vi "createActuator.vi"(8 "error in (no error)":errorcluster, 10 "Actuator Types":T1, 11 "IActuatorFactory in":refnum<class "ActuatorFactory.lvclass">) -> (0 "error out":errorcluster, 2 "Actuator":refnum<class "IActuator.lvclass">, 3 "IActuatorFactory out":refnum<class "ActuatorFactory.lvclass">)   [LabVIEW 2015, in "ActuatorFactory.lvclass"]
uses:
  ActuatorFactory.lvclass
  IActuator/IActuator.lvclass
  Typedefs/Actuator Types.ctl
  Typedefs/Pressure Servo Settings.ctl
  Typedefs/ClosedLoopSettings.ctl
  Typedefs/Flow Control Settings.ctl
  Typedefs/DAC Settings.ctl
  Calculators/VoltageToILCDACRaw/VoltageToILCDACRaw.lvclass
  ActuatorCylinder/ILCControlledActuatorCylinder/ILCControlledActuatorCylinder.lvclass
  ILCDACFactory/ILCDACFactory/ILCDACFactory.lvclass
  Calculators/VoltageToILCDACRaw/VoltageToILCDACRaw.lvclass/VoltageToILCDACRaw.ctl
  ActuatorCylinder/ILCControlledActuatorCylinder/ILCControlledActuatorCylinder.lvclass/ILCControlledActuatorCylinder.ctl
  SingleCylinderActuator/SingleCylinderActuator.lvclass
  SingleCylinderActuator/SingleCylinderActuator.lvclass/SingleCylinderActuator.ctl
  ConfigurationTestParameters/ConfigurationTestParameters.lvclass
  Typedefs/FAMTTypedefs.lvlib
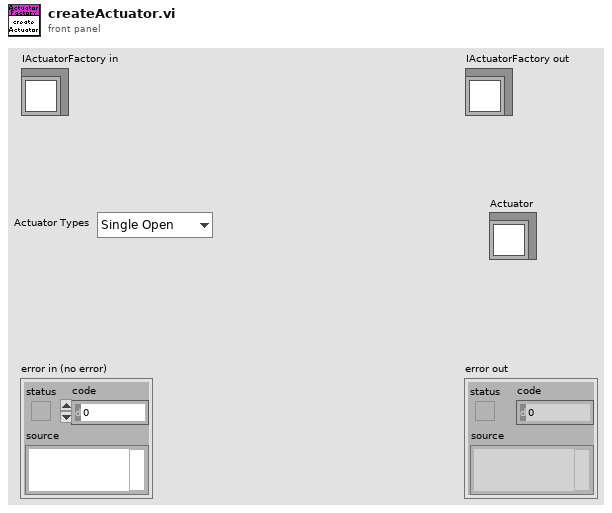
[diagram p1: front panel]
types:
  T1 = typedef "FAMTTypedefs.lvlib/Actuator Types.ctl" = enum16{"Single Open"}
  T2 = typedef "FAMTTypedefs.lvlib/DAC Settings.ctl" = cluster{"Voltage Reference":dbl[unit], "Min Counts":i32, "Max Counts":i32}
  T3 = typedef "FAMTTypedefs.lvlib/Flow Control Settings.ctl" = cluster{"DAC Channel":u8, "ROT Bias":u8, "Minimum Voltage":dbl, "Maximum Voltage":dbl, "Off Value":dbl}
  T4 = typedef "FAMTTypedefs.lvlib/Pressure Servo Settings.ctl" = cluster{"Center Point":dbl[unit], "Area":dbl, "PA to PSI":dbl, "Servo 1 DAC Channel":u8, "Servo 2 DAC Channel":u8, "Closed Loop Settings":T5, "Off Value":dbl}
  T5 = typedef "FAMTTypedefs.lvlib/ClosedLoopSettings.ctl" = cluster{"P":dbl, "I":dbl, "D":dbl, "Minimum":dbl, "Maximum":dbl}
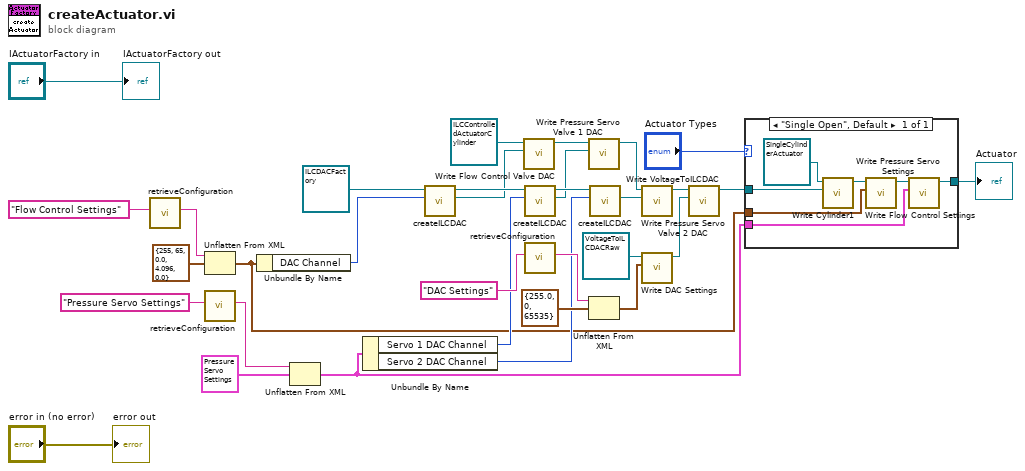
[diagram p0: block diagram]
diagram:
  n1 = call "retrieveConfiguration.vi"("configName"="Flow Control Settings") -> ("xmlConfig"=w25:string)  [unwired: 8 in, 2 out]
  n2 = Unflatten From XML(xml string=w25, type=T3 {"DAC Channel"=255, "ROT Bias"=65, "Minimum Voltage"=0.0, "Maximum Voltage"=4.096, "Off Value"=0.0} ("Flow Control Settings")) -> (value=w1:T3)  [unwired: 1 in, 1 out]
  n3 = call "retrieveConfiguration.vi"("configName"="Pressure Servo Settings") -> ("xmlConfig"=w28:string)  [unwired: 8 in, 2 out]
  n4 = Unbundle By Name(w1) -> ("DAC Channel"=w6:u8)
  n5 = Unflatten From XML(xml string=w28, type=T4 {"Center Point"=413685.4733709468, "Area"=0.004536, "PA to PSI"=0.000145038, "Servo 1 DAC Channel"=1, "Servo 2 DAC Channel"=2, "Closed Loop Settings"={"P"=1.0, "I"=0.1, "D"=0.0, "Minimum"=0.0, "Maximum"=10.0}, "Off Value"=0.004536} ("Pressure Servo Settings")) -> (value=w4:T4)  [unwired: 1 in, 1 out]
  n6 = Unbundle By Name(w4) -> ("Servo 1 DAC Channel"=w15:u8, "Servo 2 DAC Channel"=w14:u8)
  n7 = call-dynamic "createILCDAC.vi"("Channel"=w6, "ILCDACFactory in"=refnum<class "ILCDACFactory.lvclass"> refnum ("ILCDACFactory.lvclass")) -> ("ILCDAC"=w5:refnum<class "IILCDAC.lvclass">, "ILCDACFactory out"=w17:refnum<class "ILCDACFactory.lvclass">)  [unwired: 7 in, 1 out]
  n8 = call "Write Flow Control Valve DAC.vi"("IILCDAC"=w5, "ILCControlledActuatorCylinder in"=refnum<class "ILCControlledActuatorCylinder.lvclass"> refnum ("ILCControlledActuatorCylinder.lvclass")) -> ("ILCControlledActuatorCylinder out"=w8:refnum<class "ILCControlledActuatorCylinder.lvclass">)  [unwired: 9 in]
  n9 = call-dynamic "createILCDAC.vi"("Channel"=w15, "ILCDACFactory in"=w17) -> ("ILCDAC"=w13:refnum<class "IILCDAC.lvclass">, "ILCDACFactory out"=w16:refnum<class "ILCDACFactory.lvclass">)  [unwired: 7 in, 1 out]
  n10 = call "retrieveConfiguration.vi"("configName"="DAC Settings") -> ("xmlConfig"=w22:string)  [unwired: 8 in, 2 out]
  n11 = call "Write Pressure Servo Valve 1 DAC.vi"("IILCDAC"=w13, "ILCControlledActuatorCylinder in"=w8) -> ("ILCControlledActuatorCylinder out"=w11:refnum<class "ILCControlledActuatorCylinder.lvclass">)  [unwired: 9 in]
  n12 = Unflatten From XML(xml string=w22, type=T2 {"Voltage Reference"=255.0, "Min Counts"=0, "Max Counts"=65535} ("DAC Settings")) -> (value=w20:T2)  [unwired: 1 in, 1 out]
  n13 = call-dynamic "createILCDAC.vi"("Channel"=w14, "ILCDACFactory in"=w16) -> ("ILCDAC"=w12:refnum<class "IILCDAC.lvclass">)  [unwired: 7 in, 2 out]
  n14 = call "Write Pressure Servo Valve 2 DAC.vi"("IILCDAC"=w12, "ILCControlledActuatorCylinder in"=w11) -> ("ILCControlledActuatorCylinder out"=w10:refnum<class "ILCControlledActuatorCylinder.lvclass">)  [unwired: 9 in]
  n15 = call "Write DAC Settings.vi"("DAC Settings"=w20, "VoltageToILCDACRaw in"=refnum<class "VoltageToILCDACRaw.lvclass"> refnum ("VoltageToILCDACRaw.lvclass")) -> ("VoltageToILCDACRaw out"=w9:refnum<class "VoltageToILCDACRaw.lvclass">)  [unwired: 9 in]
  n16 = call "Write VoltageToILCDAC.vi"("VoltageToILCDAC"=w9, "ILCControlledActuatorCylinder in"=w10) -> ("ILCControlledActuatorCylinder out"=w3:refnum<class "ILCControlledActuatorCylinder.lvclass">)  [unwired: 9 in]
  n17 = case shown="\"Single Open\", Default" "Actuator Types" {
    tunnel: w4 -> [w39]
    tunnel: w3 -> [w37]
    tunnel: [w33] -> w2
    tunnel: w1 -> [w38]
    frame "Single Open", Default {
      n18 = call "Write Cylinder1.vi"("IActuatorCylinder.lvclass"=w37, "SingleCylinderActuator in"=refnum<class "SingleCylinderActuator.lvclass"> refnum ("SingleCylinderActuator.lvclass")) -> ("SingleCylinderActuator out"=w35:refnum<class "SingleCylinderActuator.lvclass">)  [unwired: 9 in]
      n19 = call "Write Flow Control Settings.vi"("Flow Control Settings"=w38, "SingleCylinderActuator in"=w35) -> ("SingleCylinderActuator out"=w34:refnum<class "SingleCylinderActuator.lvclass">)  [unwired: 9 in]
      n20 = call "Write Pressure Servo Settings.vi"("Pressure Servo Settings"=w39, "SingleCylinderActuator in"=w34) -> ("SingleCylinderActuator out"=w33:refnum<class "SingleCylinderActuator.lvclass">)  [unwired: 9 in]
    }
  }
  "Actuator" <- w2
  "error out" <- "error in (no error)"
  "IActuatorFactory out" <- "IActuatorFactory in"
